vi "Testbed Detection Logic.vi"() -> ()   [LabVIEW 2026]
uses:
  <extravilib>/ChannelInstances/Tag-bool/Read With Abort.vi
  <extravilib>/ChannelInstances/Tag-bool/Write With Abort.vi
  <extravilib>/ChannelInstances/Tag-bool/Instantiate.vi
  <extravilib>/ChannelInstances/Tag-bool/EndpointRead.vi
  <extravilib>/ChannelInstances/Tag-bool/Endpoint.vi
  <extravilib>/ChannelInstances/Tag-bool.lvlib
panel:
  out "Multiplier":u16
  in  "Random Number Max":u8=20
  out "Random Number":u8
  out "Score":u16
  in  "Speed Threshold, ticks":u64=3000
  in  "stop":bool
  in  "Pressed":bool[](array[boolean])
  out "Valid":bool[](array[boolean])
  in  "Random Count":i32
  in  "Debounce Threshold, ticks":u64=3000
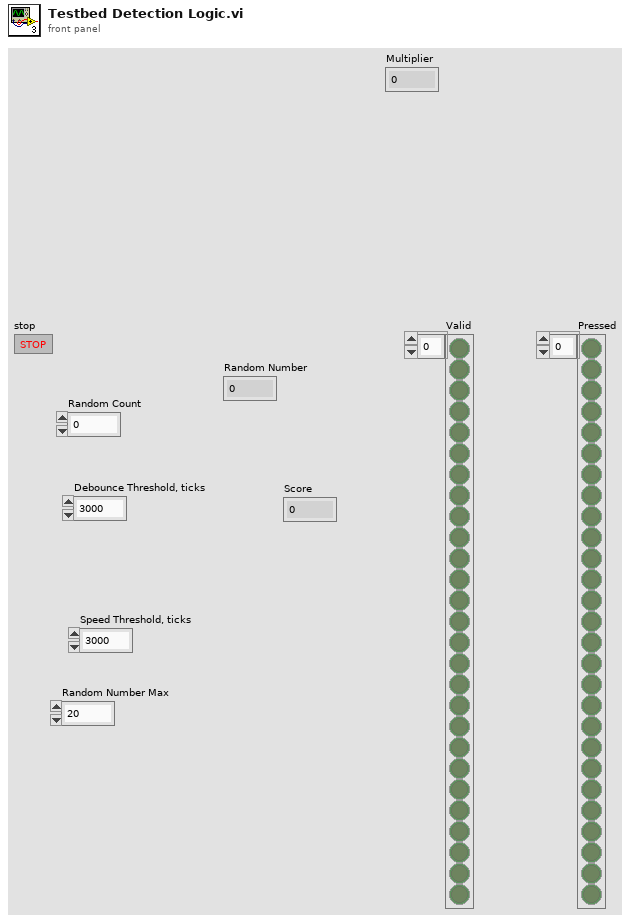
[diagram p1: front panel]
types:
  T1 = typedef "Tag-bool.lvlib/))Channel.ctl" = refnum<queue>
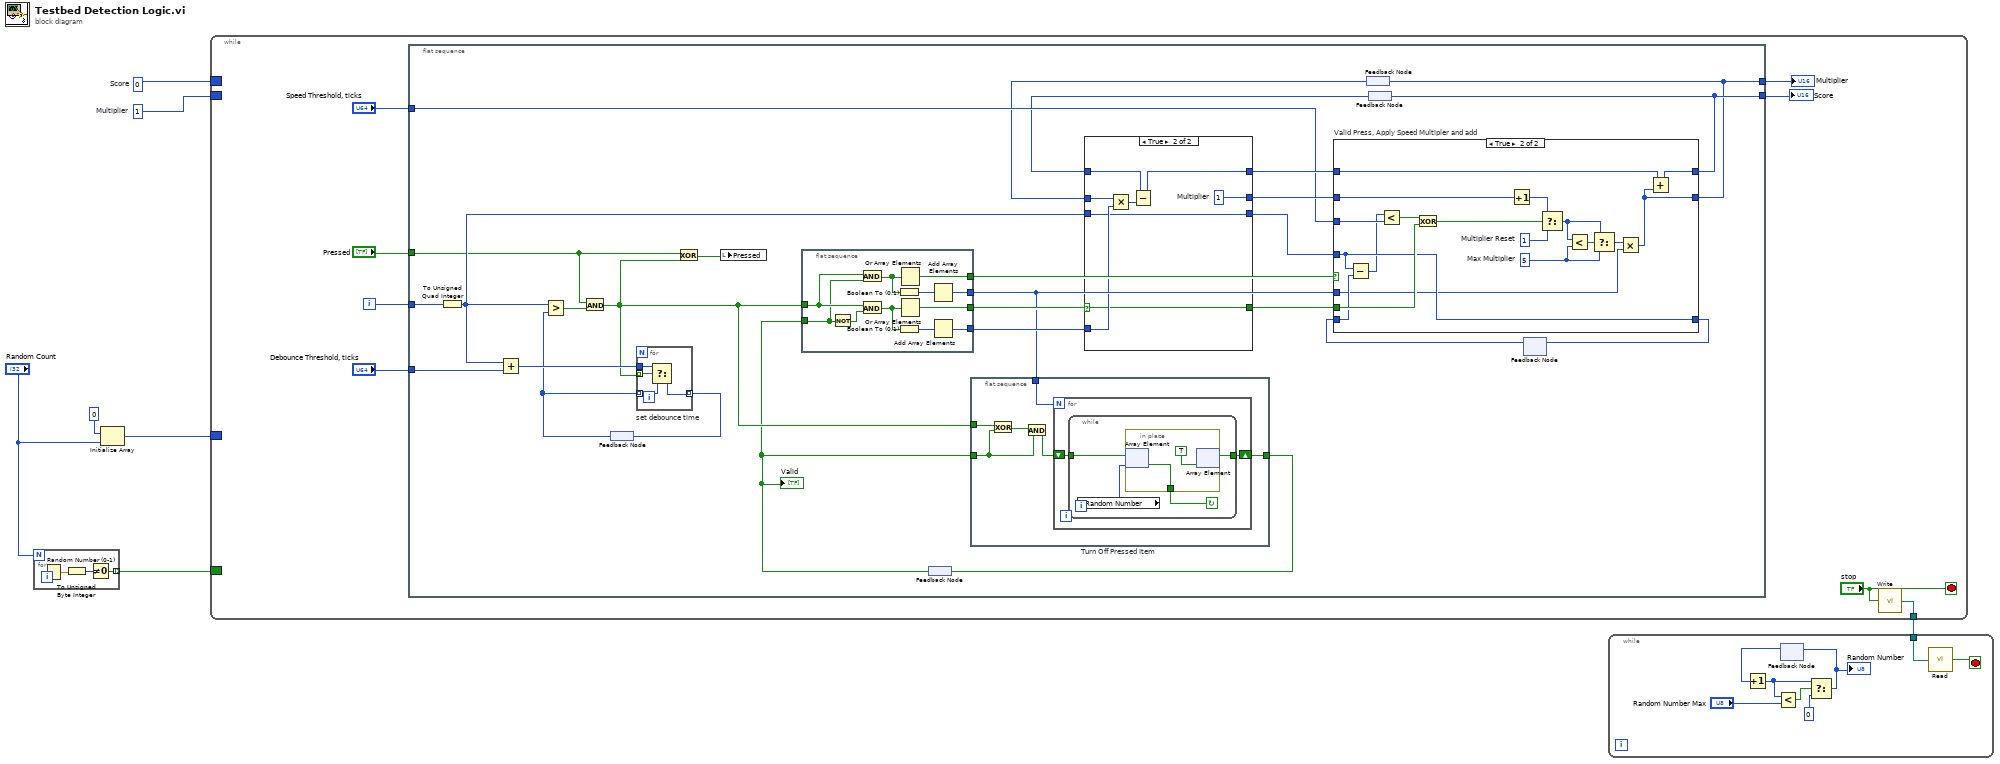
[diagram p0: block diagram]
diagram:
  w3 = u16 0  # Score
  w2 = u16 1  # Multiplier
  n1 = for {
    N: "Random Count" -> [_]
    tunnel: [w8] -> w4 mode=indexing
    n2 = Random Number (0-1)() -> (number: 0 to 1=w10:dbl)
    n3 = To Unsigned Byte Integer(number=w10) -> (unsigned 8bit integer=w9:u8)
    n4 = Not Equal To 0?(x=w9) -> (x != 0?=w8:bool)
  }
  n5 = Initialize Array(u64 0 ("Bonus Threshold"), "Random Count") -> (w5:u64[])
  n6 = while {
    border: w5 -> [_]
    border: w4 -> [_]
    border: w2 -> [_]
    border: w3 -> [_]
    tunnel: [w12] -> w1
    i -> [w18]
    stop <- "stop" stop-if-true
    n7 = flat-sequence {
      tunnel: w18 -> [w44]
      tunnel: "Debounce Threshold, ticks" -> [w42]
      tunnel: "Speed Threshold, ticks" -> [w34]
      tunnel: "Pressed" -> [w28]
      tunnel: [w24] -> w14
      tunnel: [w20] -> w11
      frame #0 {
        n8 = To Unsigned Quad Integer(1:w44) -> (0:w32:u64)
        n9 = Add(x=w32, y=w42) -> (x+y=w43:u64)
        n10 = feedback #1() -> (w39:u64[])
        n11 = Greater?(x=w32, y=w39) -> (0:w45:bool[])
        n12 = And(x=w28, y=w45) -> (x .and. y?=w25:bool[])
        n13 = for "set debounce time" {
          tunnel: w25 -> [w96] mode=indexing
          tunnel: w39 -> [w94] mode=indexing
          tunnel: w43 -> [w95]
          tunnel: [w93] -> w40 mode=indexing
          n14 = Select(t=w95, s=w96, f=w94) -> (s? t:f=w93:u64)
        }
        n15 = feedback-in #1(w40) -> ()
        n16 = Exclusive Or(1:w25, 2:w28) -> (0:w27:bool[])
        n17 = local write "Pressed"(w27) -> ()
        n18 = flat-sequence {
          tunnel: w25 -> [w107]
          tunnel: [w105] -> w38
          tunnel: w19 -> [w104]
          tunnel: [w103] -> w41
          tunnel: [w100] -> w37
          tunnel: [w97] -> w26
          frame #0 {
            n19 = Not(x=w104) -> (.not. x?=w106:bool[])
            n20 = And(x=w107, y=w104) -> (x .and. y?=w98:bool[])
            n21 = And(x=w107, y=w106) -> (x .and. y?=w102:bool[])
            n22 = Boolean To (0,1)(Boolean=w98) -> (0, 1=w99:i16[])
            n23 = Boolean To (0,1)(Boolean=w102) -> (0, 1=w101:i16[])
            n24 = Or Array Elements(Boolean array=w98) -> (logical OR=w103:bool)
            n25 = Or Array Elements(Boolean array=w102) -> (logical OR=w105:bool)
            n26 = Add Array Elements(numeric array=w99) -> (sum=w97:i16)
            n27 = Add Array Elements(numeric array=w101) -> (sum=w100:i16)
          }
        }
        n28 = feedback #2() -> (w19:bool[])
        "Valid" <- w19
        n29 = feedback-in #2(w22) -> ()
        n30 = flat-sequence "Turn Off Pressed Item" {
          tunnel: w25 -> [w49]
          tunnel: [w48] -> w22
          tunnel: w19 -> [w50]
          tunnel: w26 -> [w46]
          frame #0 {
            n31 = Exclusive Or(1:w50, 2:w49) -> (0:w51:bool[])
            n32 = And(x=w51, y=w50) -> (x .and. y?=w47:bool[])
            n33 = for {
              N: w46 -> [_]
              shift-right: [w52] -> w48
              shift-left: w47 -> [w53]
              n34 = while {
                tunnel: w53 -> [w57]
                tunnel: [w54] -> w52
                stop <- w55 continue-if-true
                n35 = local read "Random Number"() -> (w56:u8)
                n36 = in-place {
                  in-place-border: [w59] -> w55
                  n37 = in-place-array #3(w57, w56) -> (w59:bool)
                  n38 = in-place-array #3(TRUE) -> (w54:bool[])  [unwired: 1 out]
                }
              }
            }
          }
        }
        n39 = feedback #4() -> (w21:u16)
        n40 = feedback #5() -> (w23:u16)
        n41 = case shown="True" w38 {
          selector: w38 -> [w60 w65]
          tunnel: w21 -> [w63 w68]
          tunnel: w32 -> [w61 w64]
          tunnel: [w63 w71] -> w35
          tunnel: w23 -> [w62 w69]
          tunnel: [w62 w70] -> w36
          tunnel: w37 -> [_ w67]
          tunnel: [w61 w64] -> w31
          tunnel: [w60 w65] -> w33
          frame False {
          }
          frame True {
            w71 = u16 1  # Multiplier
            n42 = Multiply(x=w68, y=w67) -> (x*y=w66:u16)
            n43 = Subtract(x=w69, y=w66) -> (x-y=w70:u16)
          }
        }
        n44 = feedback #6() -> (w29:u64)  [unwired: 1 in]
        n45 = case "Valid Press, Apply Speed Multipler and add" shown="True" w41 {
          tunnel: w36 -> [w73 w91]
          tunnel: w35 -> [w74 w88]
          tunnel: [w74 w75] -> w20
          tunnel: [w73 w92] -> w24
          tunnel: w34 -> [_ w90]
          tunnel: w33 -> [_ w86]
          tunnel: [w72 w85] -> w30
          tunnel: w31 -> [_ w85]
          tunnel: w29 -> [w72 w84]
          tunnel: w26 -> [_ w76]
          frame False {
          }
          frame True {
            w79 = u16 5  # Max Multiplier
            w77 = u16 1  # Multiplier Reset
            n46 = Subtract(x=w85, y=w84) -> (x-y=w83:u64)
            n47 = Less?(x=w83, y=w90) -> (x < y?=w89:bool)
            n48 = Exclusive Or(1:w86, 2:w89) -> (0:w87:bool)
            n49 = Increment(x=w88) -> (x+1=w78:u16)
            n50 = Select(t=w78, s=w87, f=w77) -> (s? t:f=w80:u16)
            n51 = Less?(x=w80, y=w79) -> (x < y?=w82:bool)
            n52 = Select(t=w80, s=w82, f=w79) -> (s? t:f=w81:u16)
            n53 = Multiply(x=w81, y=w76) -> (x*y=w75:u16)
            n54 = Add(x=w91, y=w75) -> (x+y=w92:u16)
          }
        }
        n55 = feedback-in #4(w20) -> ()
        n56 = feedback-in #5(w24) -> ()
        n57 = feedback-in #6(w30) -> ()
      }
    }
    n58 = call <extravilib>:"Write.vi"("element"="stop") -> ("channel"=w12:T1)  [unwired: 1 out]
    "Score" <- w14
    "Multiplier" <- w11
  }
  n59 = while {
    tunnel: w1 -> [w110]
    stop <- w109 stop-if-true
    n60 = feedback #7() -> (w112:u8)  [unwired: 1 in]
    n61 = Increment(x=w112) -> (x+1=w108:u8)
    n62 = Less?(x=w108, y="Random Number Max") -> (x < y?=w113:bool)
    n63 = Select(t=w108, s=w113, f=u8 0) -> (s? t:f=w115:u8)
    "Random Number" <- w115
    n64 = feedback-in #7(w115) -> ()
    n65 = call <extravilib>:"Read.vi"("channel"=w110) -> ("element"=w109:bool)  [unwired: 1 in, 1 out]
  }
